vi "Get_Channel_Map.vi"(2 "error in":errorcluster, 3 "Get default(?)":bool=TRUE, 4 "File Path":path=path "C:/Users/Daniel/Desktop/LabView/QST/Config_Files/project_reference_default.ini") -> (0 "error out":errorcluster, 1 "Channels map":T1[](array[typedef]))   [LabVIEW 2021]
uses:
  Channel_Cluster.ctl
  <vilib>/Utility/config.llb/Read Key (U32).vi
  Channel_Map_Global.vi
  <vilib>/Utility/config.llb/NI_LVConfig.lvlib
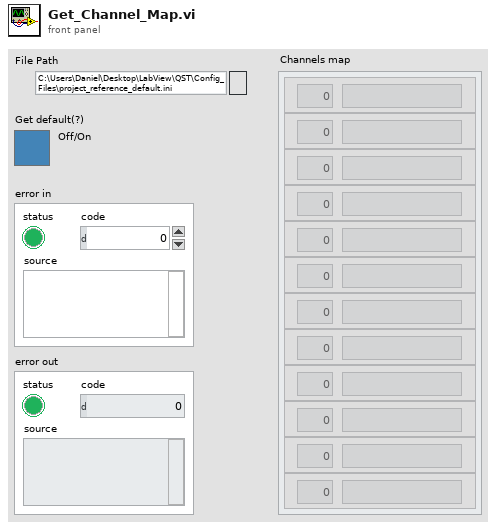
[diagram p1: front panel]
types:
  T1 = typedef "Channel_Cluster.ctl" = cluster{"Channel name":string, "Channel":u8}
  T2 = typedef "NI_LVConfig.lvlib/Config Data RefNum.ctl" = refnum<k1>
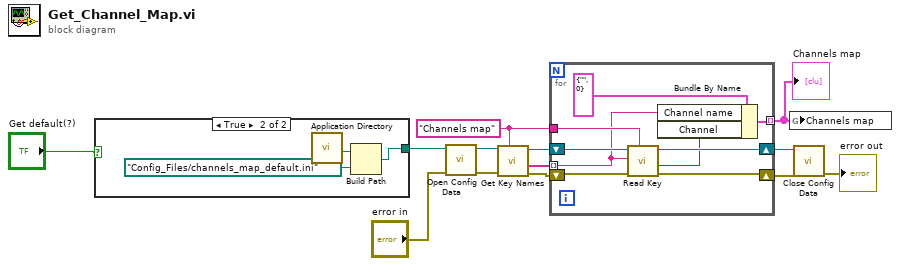
[diagram p0: block diagram]
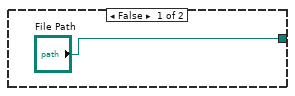
[diagram p2: hidden frame]
diagram:
  w7 = "Channels map" ("section")
  n1 = case shown="True" "Get default(?)" {
    tunnel: ["File Path" w15] -> w13
    frame False {
    }
    frame True {
      n2 = call <vilib>:"Application Directory.vi"() -> ("Application Directory"=w17:path)
      n3 = Build Path(base path=w17, name or relative path=path "Config_Files/channels_map_default.ini") -> (appended path=w15:path)
    }
  }
  n4 = call <vilib>:"Open Config Data.vi"("error in (no error)"="error in", "configuration file path"=w13) -> ("error out"=w11:errorcluster, "refnum"=w10:T2)  [unwired: 7 in, 1 out]
  n5 = call <vilib>:"Get Key Names.vi"("section"=w7, "error in (no error)"=w11, "refnum"=w10) -> ("error out"=w6:errorcluster, "key names"=w9:string[], "refnum out"=w8:T2)  [unwired: 5 in, 1 out]
  n6 = for {
    tunnel: w9 -> [w19] mode=indexing
    shift-right: [w25] -> w5
    shift-left: w8 -> [w26]
    tunnel: w7 -> [w24]
    shift-right: [w22] -> w4
    shift-left: w6 -> [w23]
    tunnel: [w18] -> w1 mode=indexing
    n7 = call-poly <vilib>:"Read Key.vi"("section"=w24, "error in (no error)"=w23, "key"=w19, "refnum"=w26) -> ("error out"=w22:errorcluster, "value"=w20:u32, "refnum out"=w25:T2)  [unwired: 4 in, 1 out]
    n8 = Bundle By Name(cluster=T1 {"Channel name"="", "Channel"=0} ("element"), "Channel name"=w19, "Channel"=w20) -> (w18:T1)
  }
  "Channels map" <- w1
  n9 = global write "Channel_Map_Global.vi" "Channels map"(w1) -> ()
  n10 = call <vilib>:"Close Config Data.vi"("error in (no error)"=w4, "refnum"=w5) -> ("error out"=→"error out":errorcluster)  [unwired: 8 in, 1 out]
